vi "mediaRobos_v2.vi"(8 "cameras array":dbl[](array[numeric]), 9 "Check Cameras?":bool=TRUE, 10 "Field Size 2":T2, 11 "Array Robot Pose + CamID":T1(array[cluster])) -> (3 "Array":cluster{"x":dbl, "y":dbl, "robot_id":i32}[](array[cluster]))   [LabVIEW 2018]
panel:
  out "Array 2":u32[][](array[numeric])
  in  "Cam Intersection Widht":u32=6
  in  "Cam Intersection Lenght":u32=6
  in  "file path (use dialog) 2":path=path "C:/Users/RoboIme/git/sslview/Util/Farias2.csv"
  in  "cluster":cluster{"x":dbl, "y":dbl, "robot_id":i32}
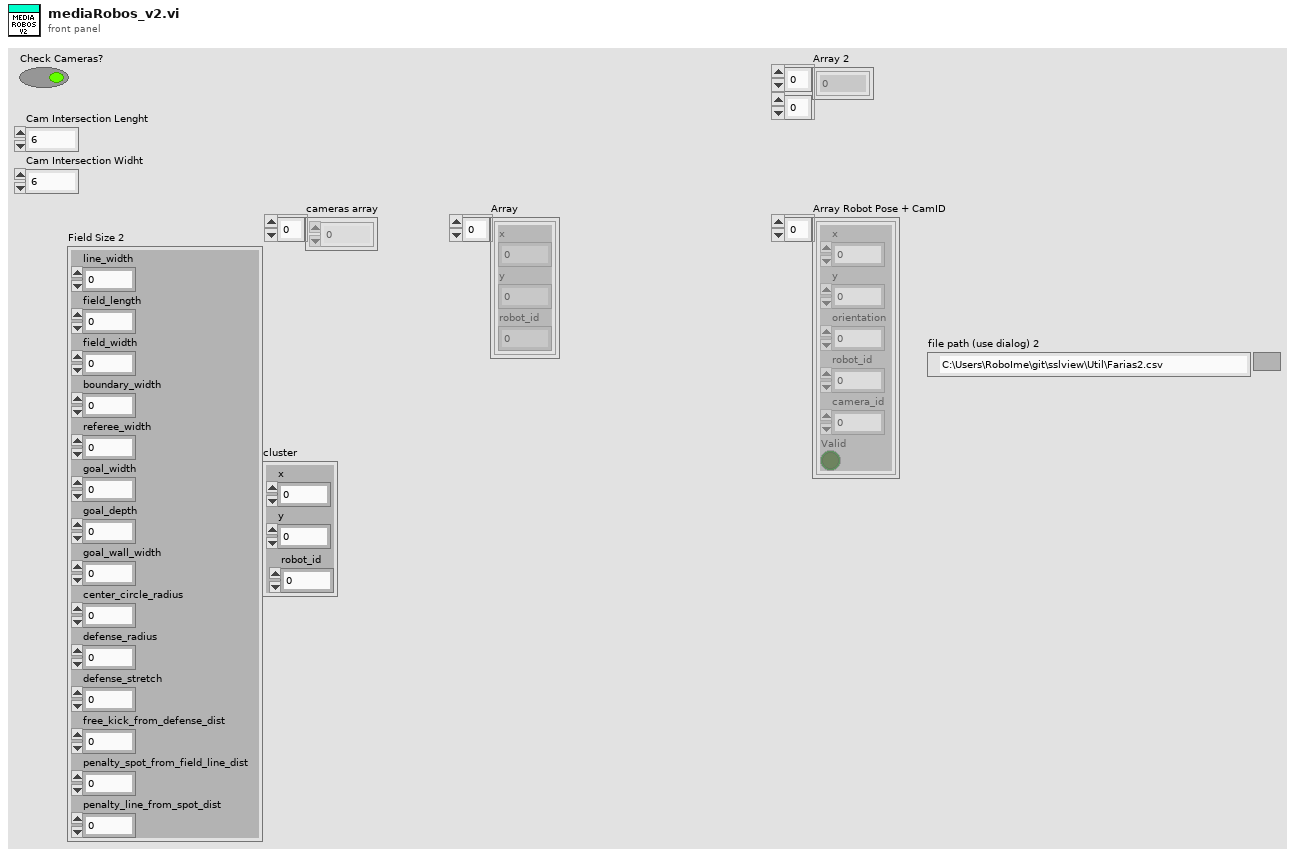
[diagram p1: front panel]
types:
  T1 = cluster{"x":sgl, "y":sgl, "orientation":sgl, "robot_id":u32, "camera_id":u32, "Valid":bool}[]
  T2 = cluster{"line_width":u32, "field_length":u32, "field_width":u32, "boundary_width":u32, "referee_width":u32, "goal_width":u32, "goal_depth":u32, "goal_wall_width":u32, "center_circle_radius":u32, "defense_radius":u32, "defense_stretch":u32, "free_kick_from_defense_dist":u32, "penalty_spot_from_field_line_dist":u32, "penalty_line_from_spot_dist":u32}
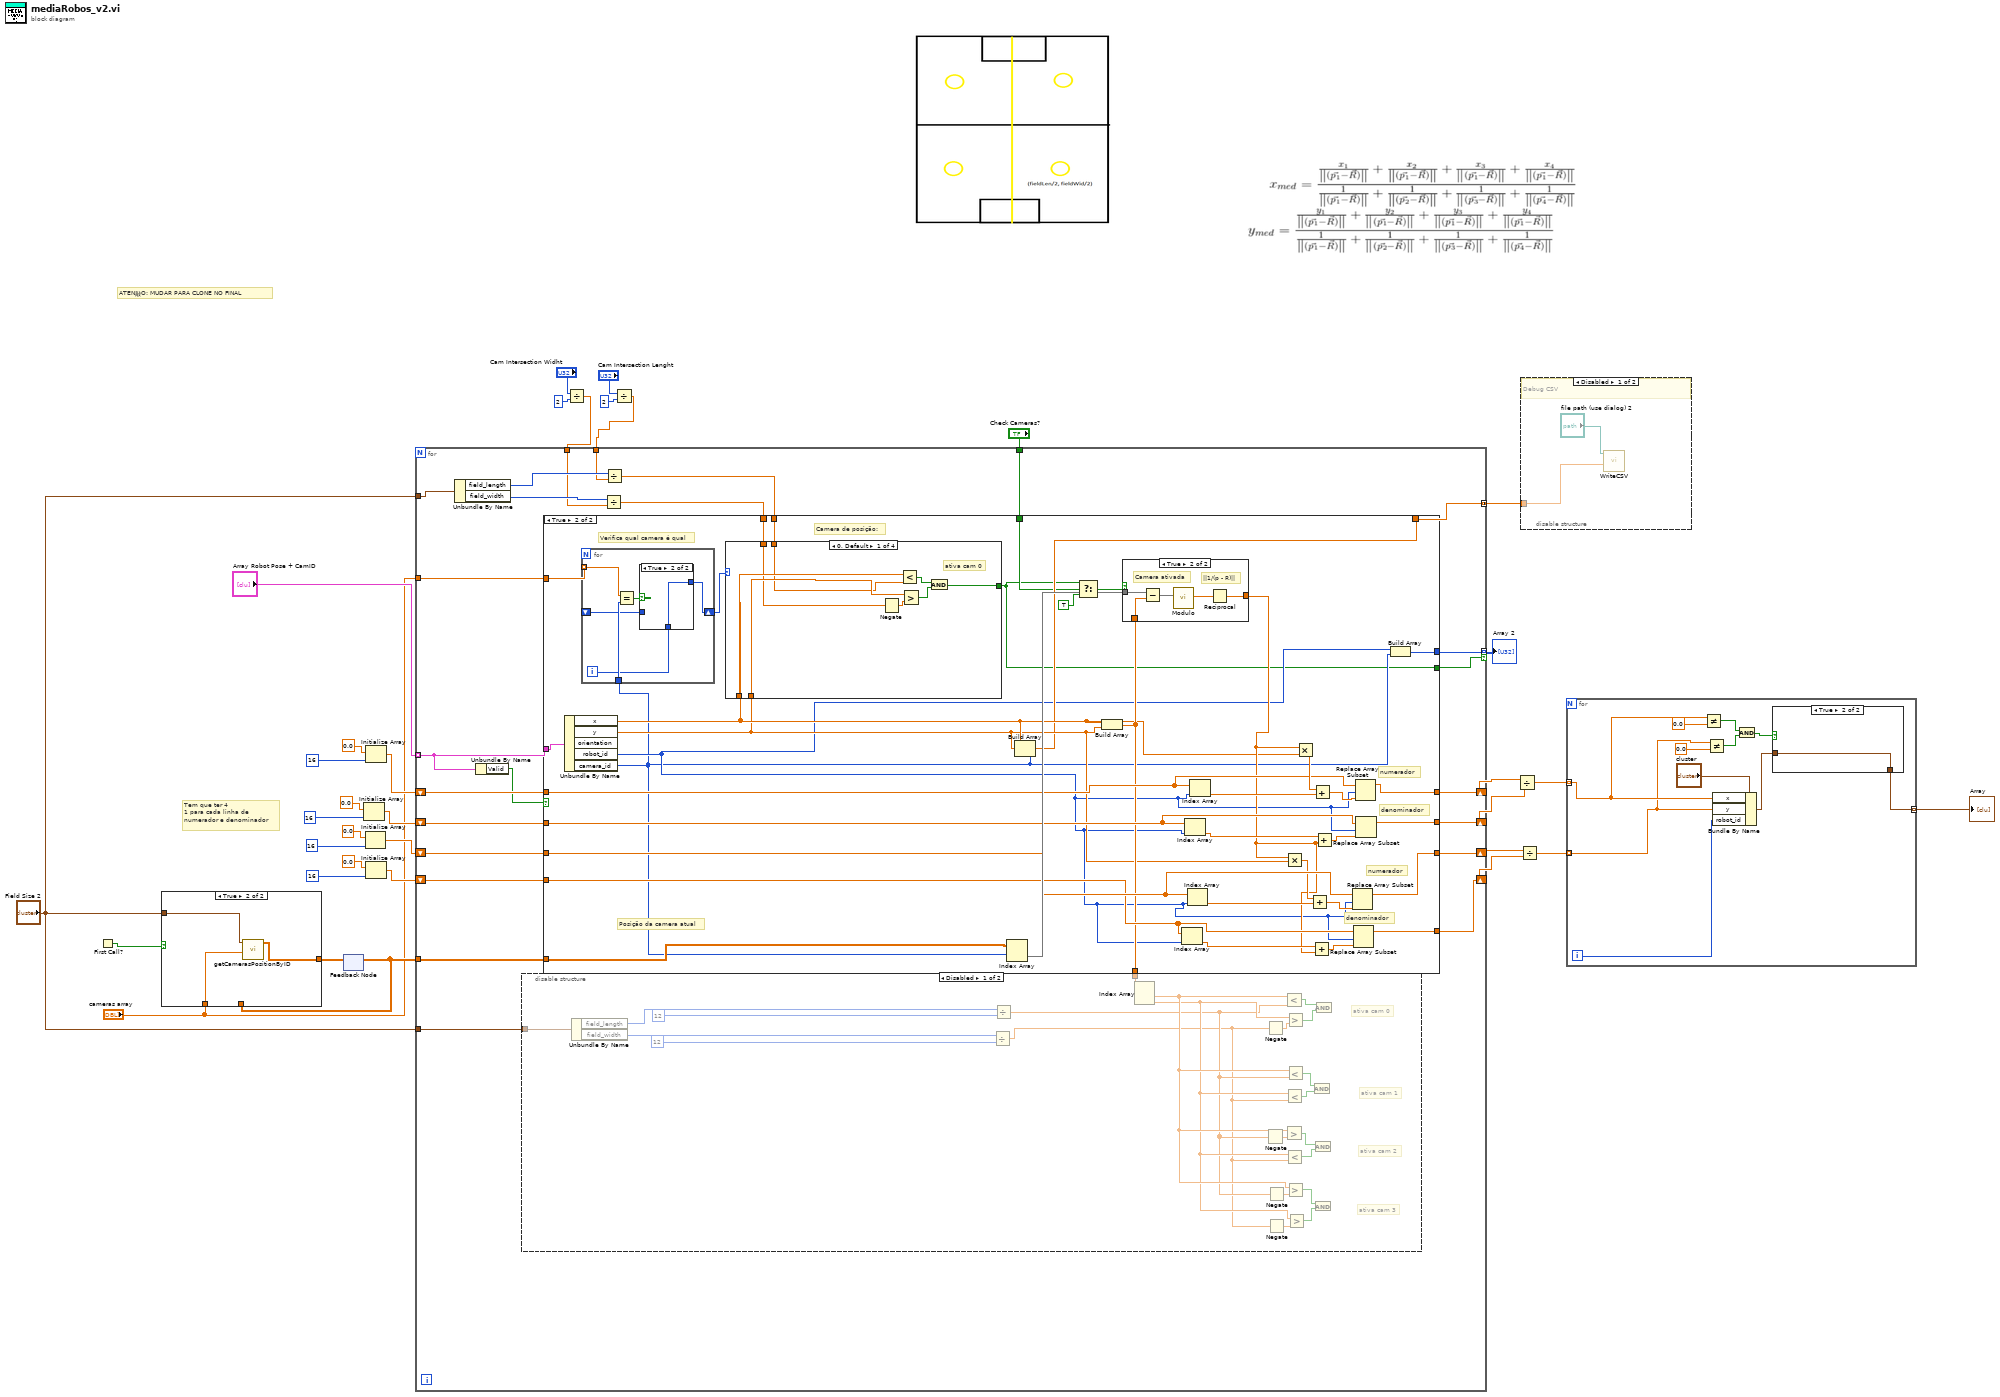
[diagram p0: block diagram]
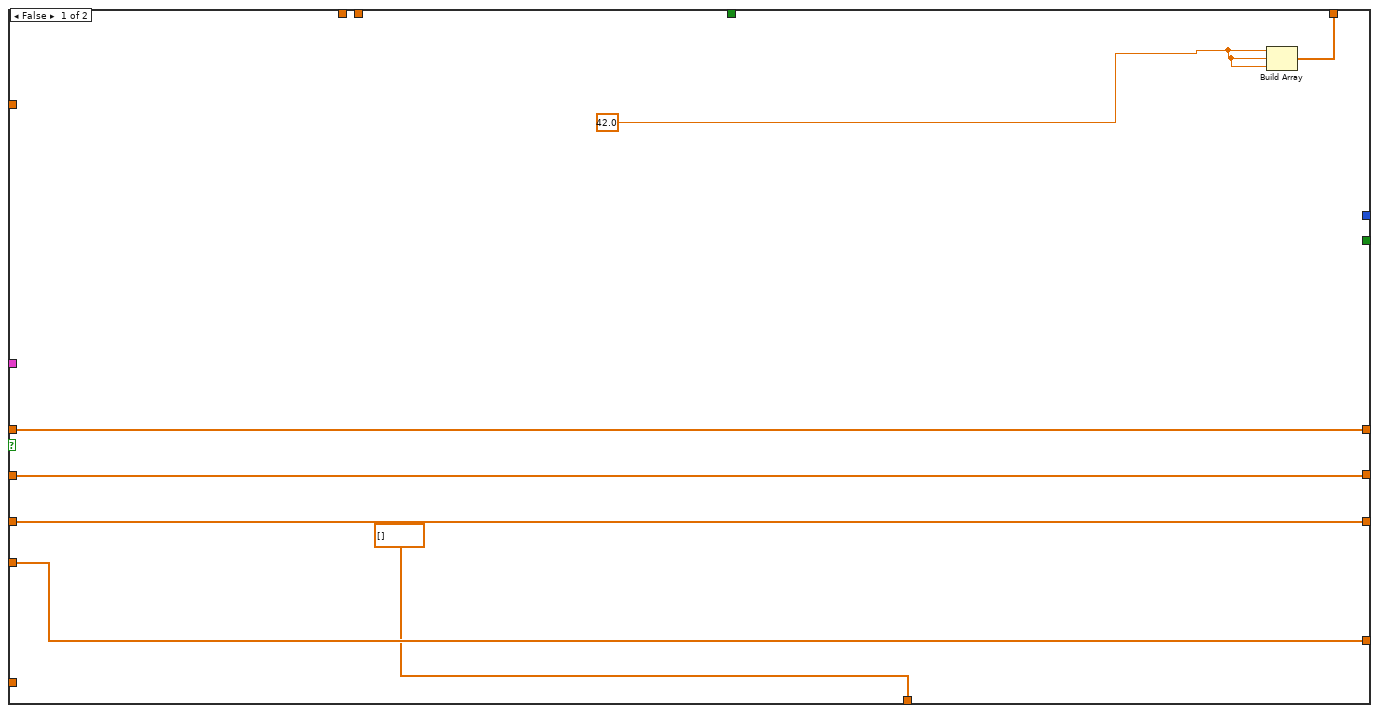
[diagram p4: hidden frame]
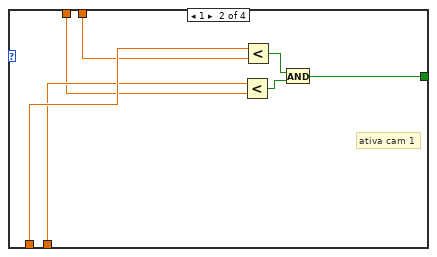
[diagram p5: hidden frame]
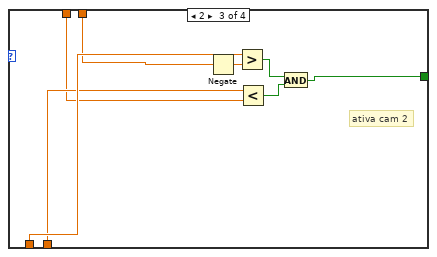
[diagram p6: hidden frame]
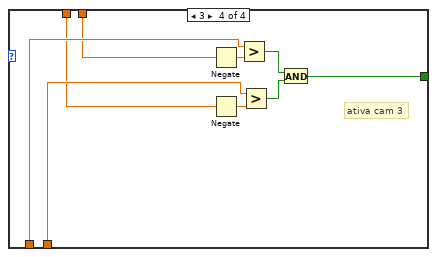
[diagram p7: hidden frame]
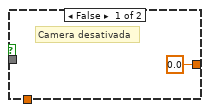
[diagram p9: hidden frame]
diagram:
  # "Tem que ter 4\n1 para cada linha de\nnumerador e denominador"
  # "ATEN敲O: MUDAR PARA CLONE NO FINAL"
  n1 = First Call?() -> (First Call?: T/F=w13:bool)
  n2 = feedback #1() -> (w11:dbl[][])  [unwired: 1 in]
  n3 = case shown="True" w13 {
    tunnel: "Field Size 2" -> [_ w38]
    tunnel: [w35 w37] -> w12
    tunnel: w11 -> [w35 _]
    tunnel: "cameras array" -> [_ w36]
    frame False {
    }
    frame True {
      n4 = call "getCamerasPositionByID.vi"("cameras id"=w36, "Field Size 2"=w38) -> ("Cameras Positions"=w37:dbl[][])  [unwired: 9 in]
    }
  }
  n5 = feedback-in #1(w12) -> ()
  n6 = Initialize Array(0.0 ("element"), 16 ("dimension size")) -> (w25:dbl[])
  n7 = Initialize Array(0.0 ("element"), 16 ("dimension size")) -> (w24:dbl[])
  n8 = Initialize Array(0.0 ("element"), 16 ("dimension size")) -> (w26:dbl[])
  n9 = Initialize Array(0.0 ("element"), 16 ("dimension size")) -> (w23:dbl[])
  n10 = Divide(x="Cam Intersection Widht", y=u32 2) -> (x/y=w4:dbl)
  n11 = Divide(x="Cam Intersection Lenght", y=u32 2) -> (x/y=w7:dbl)
  n12 = for {
    tunnel: "Array Robot Pose + CamID" -> [w53] mode=indexing
    tunnel: w11 -> [w63]
    shift-right: [w62] -> w22
    shift-left: w26 -> [w56]
    shift-right: [w61] -> w21
    shift-left: w25 -> [w55]
    shift-right: [w60] -> w20
    shift-left: w24 -> [w58]
    shift-right: [w59] -> w19
    shift-left: w23 -> [w57]
    tunnel: [w54] -> w15 mode=concatenating
    tunnel: "Field Size 2" -> [w51]
    tunnel: "Field Size 2" -> [w49]
    tunnel: w7 -> [w44]
    tunnel: w4 -> [w43]
    tunnel: "cameras array" -> [w42]
    tunnel: "Check Cameras?" -> [w41]
    tunnel: [w40] -> w1 mode=indexing if=w39
    n13 = Unbundle By Name(w49) -> ("field_length"=w48:u32, "field_width"=w47:u32)
    n14 = Unbundle By Name(w53) -> ("Valid"=w52:bool)
    n15 = Divide(x=w47, y=w43) -> (x/y=w45:dbl)
    n16 = Divide(x=w48, y=w44) -> (x/y=w46:dbl)
    n17 = case shown="True" w52 {
      tunnel: w53 -> [_ w129]
      tunnel: w63 -> [_ w128]
      tunnel: [w92 w117] -> w62
      tunnel: [w91 w116] -> w61
      tunnel: [w90 w115] -> w60
      tunnel: [w89 w114] -> w59
      tunnel: w58 -> [w90 w113]
      tunnel: w57 -> [w89 w112]
      tunnel: w56 -> [w92 w111]
      tunnel: w55 -> [w91 w110]
      tunnel: [w88 w100] -> w54
      tunnel: [sgl[] [] w107] -> w50
      tunnel: w42 -> [_ w104]
      tunnel: w46 -> [_ w102]
      tunnel: w45 -> [_ w101]
      tunnel: w41 -> [_ w99]
      tunnel: [_ w94] -> w40
      tunnel: [_ w93] -> w39
      frame False {
        w87 = 42.0 ("element")
        n18 = Build Array(w87, w87, w87) -> (w88:dbl[])
      }
      frame True {
        # "Verifica qual camera é qual"
        # "Camera de posição:"
        # "denominador"
        # "numerador"
        # "denominador"
        # "numerador"
        # "Posição da camera atual"
        n19 = Unbundle By Name(w129) -> ("x"=w106:sgl, "y"=w105:sgl, "robot_id"=w96:u32, "camera_id"=w95:u32)  [unwired: 1 out]
        n20 = for {
          tunnel: w104 -> [w166] mode=indexing
          tunnel: w95 -> [w167]
          shift-right: [w163] -> w103
          shift-left: _ -> [w162]
          i -> [w164]
          n21 = Equal?(x=w166, y=w167) -> (x = y?=w165:bool)
          n22 = case shown="True" w165 {
            tunnel: w164 -> [_ w169]
            tunnel: [w168 w169] -> w163
            tunnel: w162 -> [w168 _]
            frame False {
            }
            frame True {
            }
          }
        }
        n23 = case shown="0, Default" w103 {
          tunnel: w106 -> [w134 w142 w149 w157]
          tunnel: w105 -> [w133 w141 w148 w156]
          tunnel: [w130 w138 w145 w153] -> w93
          tunnel: w102 -> [w132 w140 w147 w155]
          tunnel: w101 -> [w131 w139 w146 w154]
          frame 0, Default {
            # "ativa cam 0"
            n24 = Negate(x=w131) -> (-x=w135:dbl)
            n25 = Less?(x=w134, y=w132) -> (x < y?=w137:bool)
            n26 = Greater?(x=w133, y=w135) -> (0:w136:bool)
            n27 = And(x=w137, y=w136) -> (x .and. y?=w130:bool)
          }
          frame 1 {
            # "ativa cam 1"
            n28 = Less?(x=w141, y=w139) -> (x < y?=w144:bool)
            n29 = Less?(x=w142, y=w140) -> (x < y?=w143:bool)
            n30 = And(x=w143, y=w144) -> (x .and. y?=w138:bool)
          }
          frame 2 {
            # "ativa cam 2"
            n31 = Negate(x=w147) -> (-x=w152:dbl)
            n32 = Greater?(x=w149, y=w152) -> (0:w151:bool)
            n33 = Less?(x=w148, y=w146) -> (x < y?=w150:bool)
            n34 = And(x=w151, y=w150) -> (x .and. y?=w145:bool)
          }
          frame 3 {
            # "ativa cam 3"
            n35 = Negate(x=w155) -> (-x=w161:dbl)
            n36 = Negate(x=w154) -> (-x=w160:dbl)
            n37 = Greater?(x=w157, y=w161) -> (0:w158:bool)
            n38 = Greater?(x=w156, y=w160) -> (0:w159:bool)
            n39 = And(x=w158, y=w159) -> (x .and. y?=w153:bool)
          }
        }
        n40 = Index Array(array=w128, index (row)=w95) -> (element=w122:dbl[])  [unwired: 1 in]
        n41 = Build Array(w106, w105, w95) -> (w100:sgl[])
        n42 = Select(t=w93, s=w99, f=TRUE) -> (s? t:f=w97:bool)
        n43 = Build Array(w106, w105) -> (w107:sgl[])
        n44 = case shown="True" w97 {
          tunnel: w122 -> [_ w173]
          tunnel: [0.0 w172] -> w108
          tunnel: w107 -> [_ w171]
          frame False {
            # "Camera desativada"
          }
          frame True {
            # "Camera ativada"
            # "||1/(p - R)||"
            n45 = Subtract(x=w173, y=w171) -> (x-y=w175:dbl[])
            n46 = call "Modulo.vi"("2D vector"=w175) -> ("Modulo"=w174:dbl)  [unwired: 10 in]
            n47 = Reciprocal(x=w174) -> (1/x=w172:dbl)
          }
        }
        n48 = Index Array(array=w112, index=w96) -> (element=w118:dbl)
        n49 = Index Array(array=w110, index=w96) -> (element=w120:dbl)
        n50 = Index Array(array=w113, index=w96) -> (element=w119:dbl)
        n51 = Index Array(array=w111, index=w96) -> (element=w121:dbl)
        n52 = Multiply(x=w108, y=w105) -> (x*y=w109:dbl)
        n53 = Multiply(x=w108, y=w106) -> (x*y=w127:dbl)
        n54 = Add(x=w109, y=w119) -> (x+y=w124:dbl)
        n55 = Add(x=w118, y=w108) -> (x+y=w123:dbl)
        n56 = Add(x=w127, y=w121) -> (x+y=w126:dbl)
        n57 = Add(x=w120, y=w108) -> (x+y=w125:dbl)
        n58 = Replace Array Subset(array=w113, new element=w124, index=w96) -> (w115:dbl[])
        n59 = Replace Array Subset(array=w112, new element=w123, index=w96) -> (w114:dbl[])
        n60 = Replace Array Subset(array=w111, new element=w126, index=w96) -> (w117:dbl[])
        n61 = Replace Array Subset(array=w110, new element=w125, index=w96) -> (w116:dbl[])
        n62 = Build Array(w96, w95) -> (w94:u32[])
      }
    }
    n63 = disable-structure shown="Disabled" {
      disable-tunnel: w51 -> [w85 _]
      disable-tunnel: w50 -> [w80 _]
      frame Disabled {
        # "ativa cam 3"
        # "ativa cam 2"
        # "ativa cam 1"
        # "ativa cam 0"
        n64 = Unbundle By Name(w85) -> ("field_length"=w81:u32, "field_width"=w82:u32)
        n65 = Divide(x=w82, y=u32 12) -> (x/y=w64:dbl)
        n66 = Divide(x=w81, y=u32 12) -> (x/y=w65:dbl)
        n67 = Index Array(array=w80) -> (element #1=w67:sgl, element #2=w66:sgl)  [unwired: 2 in]
        n68 = Negate(x=w65) -> (-x=w74:dbl)
        n69 = Negate(x=w64) -> (-x=w77:dbl)
        n70 = Negate(x=w65) -> (-x=w71:dbl)
        n71 = Negate(x=w64) -> (-x=w70:dbl)
        n72 = Less?(x=w67, y=w65) -> (x < y?=w79:bool)
        n73 = Greater?(x=w67, y=w74) -> (0:w73:bool)
        n74 = Less?(x=w66, y=w64) -> (x < y?=w76:bool)
        n75 = Less?(x=w66, y=w64) -> (x < y?=w72:bool)
        n76 = Greater?(x=w66, y=w77) -> (0:w78:bool)
        n77 = Less?(x=w67, y=w65) -> (x < y?=w75:bool)
        n78 = Greater?(x=w67, y=w71) -> (0:w68:bool)
        n79 = Greater?(x=w66, y=w70) -> (0:w69:bool)
        n80 = And(x=w75, y=w76) -> ()  [unwired: 1 out]
        n81 = And(x=w73, y=w72) -> ()  [unwired: 1 out]
        n82 = And(x=w68, y=w69) -> ()  [unwired: 1 out]
        n83 = And(x=w79, y=w78) -> ()  [unwired: 1 out]
      }
      frame Enabled {
      }
    }
  }
  "Array 2" <- w1
  n84 = Divide(x=w22, y=w21) -> (x/y=w18:dbl[])
  n85 = Divide(x=w20, y=w19) -> (x/y=w17:dbl[])
  n86 = disable-structure "Diagram Disable Structure" shown="Disabled" {
    disable-tunnel: w15 -> [w177 _]
    frame Disabled {
      # "Debug CSV"
      n87 = call "WriteCSV.vi"("array"=w177, "file path (use dialog)"="file path (use dialog) 2") -> ()  [unwired: 10 in]
    }
    frame Enabled {
    }
  }
  n88 = for {
    tunnel: w18 -> [w187] mode=indexing
    tunnel: w17 -> [w184] mode=indexing
    tunnel: [w180] -> w16 mode=indexing
    i -> [w188]
    n89 = Not Equal?(x=w187, y=0.0) -> (x != y?=w183:bool)
    n90 = Not Equal?(x=w184, y=0.0) -> (x != y?=w182:bool)
    n91 = Bundle By Name(cluster="cluster", "x"=w187, "y"=w184, "robot_id"=w188) -> (w179:cluster{"x":dbl, "y":dbl, "robot_id":i32})
    n92 = And(x=w183, y=w182) -> (x .and. y?=w181:bool)
    n93 = case shown="True" w181 {
      tunnel: [w189 w190] -> w180
      tunnel: w179 -> [w189 w190]
      frame False {
      }
      frame True {
      }
    }
  }
  "Array" <- w16
